vi "accept.vi"(8 "error in (no error)":errorcluster, 10 "Visitor":refnum<class "Visitor.lvclass">, 11 "Rectangle in":refnum<class "Rectangle.lvclass">) -> (0 "error out":errorcluster, 2 "String":string, 3 "Rectangle out":refnum<class "Rectangle.lvclass">)   [LabVIEW 2018, in "Rectangle.lvclass"]
uses:
  Rectangle.lvclass
  Visitor Class/Visitor.lvclass
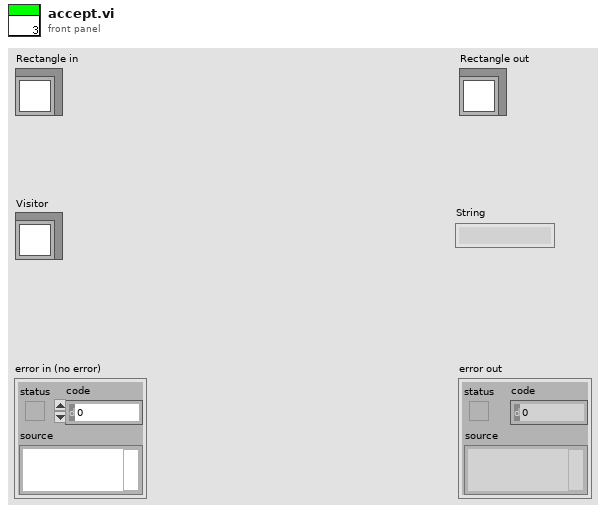
[diagram p1: front panel]
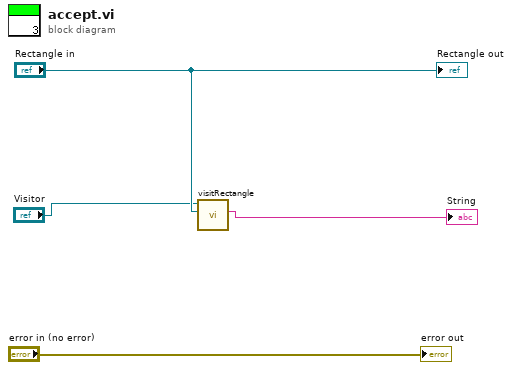
[diagram p0: block diagram]
diagram:
  n1 = call-dynamic "visitRectangle.vi"("Rectangle"="Rectangle in", "Visitor in"="Visitor") -> ("String"=→"String":string)  [unwired: 7 in, 2 out]
  "error out" <- "error in (no error)"
  "Rectangle out" <- "Rectangle in"
